vi "Interfaz.vi"() -> ()   [LabVIEW 2020]
uses:
  <vilib>/Instr/_visa.llb/Select Event Type.ctl
  <vilib>/Instr/_visa.llb/VISA Configure Serial Port (Instr).vi
panel:
  out "Temperatura > 100 °C":bool
  out "TERMOMETRO":dbl(slide) scale=0.0..100.0
  out "Temperatura en °C":string
  in  "Bytes a recibir":u32
  in  "?":u32=9600
  in  "?":refnum<visa-resource-name>
  # "ESCUELA SUPERIOR DE COMPUTO\n\nPROYECTO FINAL DE INSTRUMENTACIÓN\n\"SIMULADOR DE TEMPERATURA\"\n\nALUMNO:  HUGO ANDRES MACHORRO MELÉNDEZ\n\nGRUPO:  3CV4"
  # "Selección de puertos"
  # "Velocidad de Transmisión"
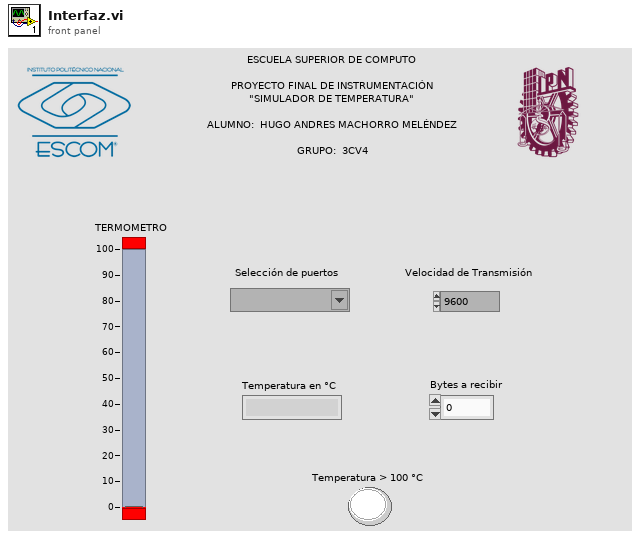
[diagram p1: front panel]
types:
  T1 = typedef "Select Event Type.ctl" = u32
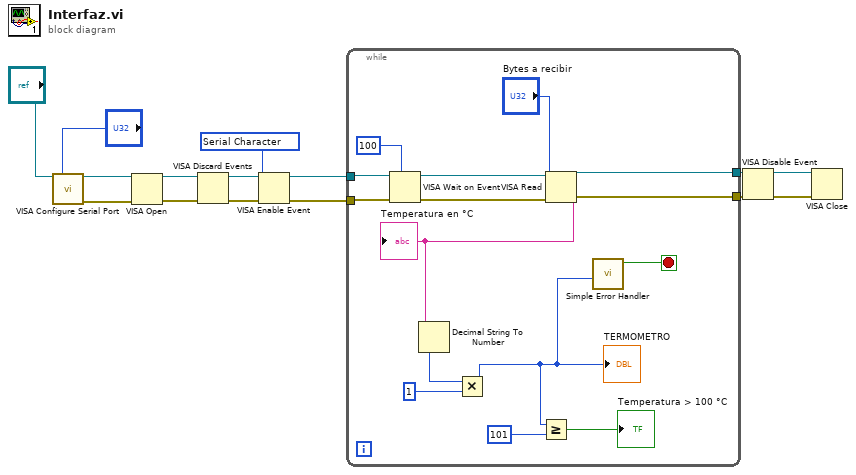
[diagram p0: block diagram]
diagram:
  w7 = T1 1073684533 items=["Service Request"=1073684491, "Trigger"=3221168138, "Clear"=1073684493, "VXI Signal"=1073684512, "VXI/VME Interrupt"=3221168161, "VXI/VME Sysfail"=1073684509, "VXI/VME Sysreset"=1073684510, "GPIB CIC"=1073684498, "GPIB Talk"=1073684499, "GPIB Listen"=1073684500, "PXI Interrupt"=1073684514, "Serial Break"=1073684515, "Serial TermChar"=1073684516, "Serial CTS"=1073684521, "Serial DSR"=1073684522, "Serial DCD"=1073684524, "Serial RI"=1073684526, "Serial Character"=1073684533, "USB Interrupt"=1073684535, "All Enabled"=1073709055] ("Event Type")
  n1 = call-poly "VISA Configure Serial Port"("VISA resource name"="?", "baud rate (9600)"="?") -> ("VISA resource name out"=w9:refnum<visa-resource-name>, "error out"=w8:errorcluster)  [unwired: 12 in]
  n2 = VISA Open(error in (no error)=w8, VISA resource name=w9) -> (VISA resource name=w11:refnum<visa-resource-name>, error out=w10:errorcluster)  [unwired: 3 in]
  n3 = VISA Discard Events(8:w10, 11:w11) -> (0:w12:errorcluster, 3:w13:refnum<visa-resource-name>)  [unwired: 2 in]
  n4 = VISA Enable Event(8:w12, 10:w7, 11:w13) -> (0:w5:errorcluster, 3:w6:refnum<visa-resource-name>)  [unwired: 1 in]
  n5 = while {
    tunnel: w6 -> [w30]
    tunnel: w5 -> [w29]
    tunnel: [w25] -> w2
    tunnel: [w17] -> w1
    stop <- w18 stop-if-true
    n6 = VISA Wait on Event(7:u32 100 ("timeout (0)"), 8:w29, 11:w30) -> (0:w28:errorcluster, 3:w27:refnum<visa-resource-name>)  [unwired: 2 in, 2 out]
    n7 = VISA Read(VISA resource name=w27, byte count="Bytes a recibir", error in (no error)=w28) -> (VISA resource name out=w25:refnum<visa-resource-name>, read buffer=w23:string, error out=w17:errorcluster)  [unwired: 1 out]
    "Temperatura en °C" <- w23
    n8 = Decimal String To Number(string=w23) -> (number=w22:i32)  [unwired: 2 in, 1 out]
    n9 = Multiply(x=w22, y=1) -> (x*y=w16:i32)
    "TERMOMETRO" <- w16
    n10 = Greater Or Equal?(x=w16, y=101 ("x")) -> (x >= y?=→"Temperatura > 100 °C":bool)
    n11 = call <vilib>:"Simple Error Handler.vi"("type of dialog (OK msg:1)"=w16) -> ("error?"=w18:bool)  [unwired: 4 in, 4 out]
  }
  n12 = VISA Disable Event(8:w1, 11:w2) -> (0:w3:errorcluster, 3:w4:refnum<visa-resource-name>)  [unwired: 2 in]
  n13 = VISA Close(VISA resource name=w4, error in (no error)=w3) -> ()  [unwired: 1 out]
